vi "F to C.vi"(11 "Fahrenheit":dbl) -> (3 "Celsius":dbl)   [LabVIEW 2013, in "Simple Dual Mode Thermometer XControl.xctl"]
doc: "This VI converts degrees Fahrenheit to degrees Celsius."
uses:
  Simple Dual Mode Thermometer XControl.xctl
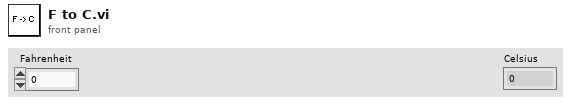
[diagram p1: front panel]
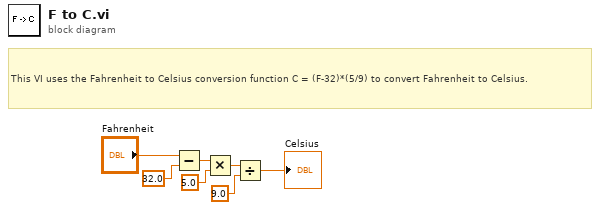
[diagram p0: block diagram]
diagram:
  # "This VI uses the Fahrenheit to Celsius conversion function C = (F-32)*(5/9) to convert Fahrenheit to Celsius."
  n1 = Subtract(x="Fahrenheit", y=32.0) -> (x-y=w7:dbl)
  n2 = Multiply(x=w7, y=5.0) -> (x*y=w6:dbl)
  n3 = Divide(x=w6, y=9.0) -> (x/y=→"Celsius":dbl)
